vi "DataTranslation_server.vi"(0 "Board type":T1=enum."DT LV-link", 1 "interval scanning":bool, 2 "Client Time":dbl=3399992102.447224, 5 "No of samples+extra":i32=200 min=0 step=1, 7 "Trigger mode":T2, 9 "output polarity":u16(ring)=1 items=["do not change", "positive", "negative"], 11 "Ch & spans":T3[](array[typedef])=[{"high limit (10V)"=10.0, "low limit (-10V)"=-10.0, "Ch No"=0, "Var name"="RV (Vin)", "Use Latest Calib"=FALSE}] {"low limit (-10V)" format="%.3f"; "high limit (10V)" format="%.3f"}, 12 "Actual Sampling rate (Hz)":dbl=10000.0 format="%.2f", 13 "Local Client?":bool=TRUE, 14 "Current Block No":i32) -> (4 "I16 data":i16[][](array[numeric]), 6 "Block Timings":T4={"Started"=3399991568.753699, "Ended"=3399991587.0837474, "Analogue Frequency Hz"=50000.0} {"Analogue Frequency Hz" format="%.2f"}, 10 "group channel settings":T5(array[cluster])=[{"channel"="", "upper input limits"=0.0, "lower input limits"=0.0, "range"=0.0, "polarity"=0, "gain"=0.0, "coupling"=0, "input mode"=0, "scale multiplier"=1.6666666666666668e-07, "scale offset"=0.0}] {"scale offset" format="%#_16f"; "scale multiplier" format="%#_16f"; "input mode" format="%#_16f"; "coupling" format="%#_16f"; "gain" format="%#_16f"; "polarity" format="%#_16f"; "range" format="%#_16f"; "lower input limits" format="%#_16f"; "upper input limits" format="%#_16f"}, 15 "error out":errorcluster={"status"=TRUE, "code"=1172, "source"="Error calling method LvLink2.LvTask.ReadDblData2DAs1D, (System.Reflection.TargetInvocationException: Exception has been thrown by the target of an invocation.\n\tInner Exception: LvLink2.LvException: Timeout) <append><b>LvLink2.LvException</b> in OLReadMultiple2D.vi->DataTranslation_server.vi->Acquire_Data.vi->Get_data.vi->Measurement.vi"})   [LabVIEW 2011]
uses:
  Controls/Block_start_and_end.ctl
  Controls/Ch_and_Spans.ctl
  Controls/Trigger_Mode.ctl
  Controls/Board_Types.ctl
  Data_Translation/DataTranslation_global.vi
  PWA/PWAtasksGLOBAL.vi
  <userlib>/LV-Link3/PolySubVIs/DtCreateAinChan.vi
  <userlib>/LV-Link3/PolySubVIs/DtOLTimingSetInput.vi
  Globals/Meas_global.vi
  <userlib>/LV-Link3/PolySubVIs/DtOLReadMultiple2D.vi
  <userlib>/LV-Link3/PolySubVIs/DtOLTriggerDigital.vi
panel:
  in  "error in":errorcluster
  out "AFG error out":errorcluster
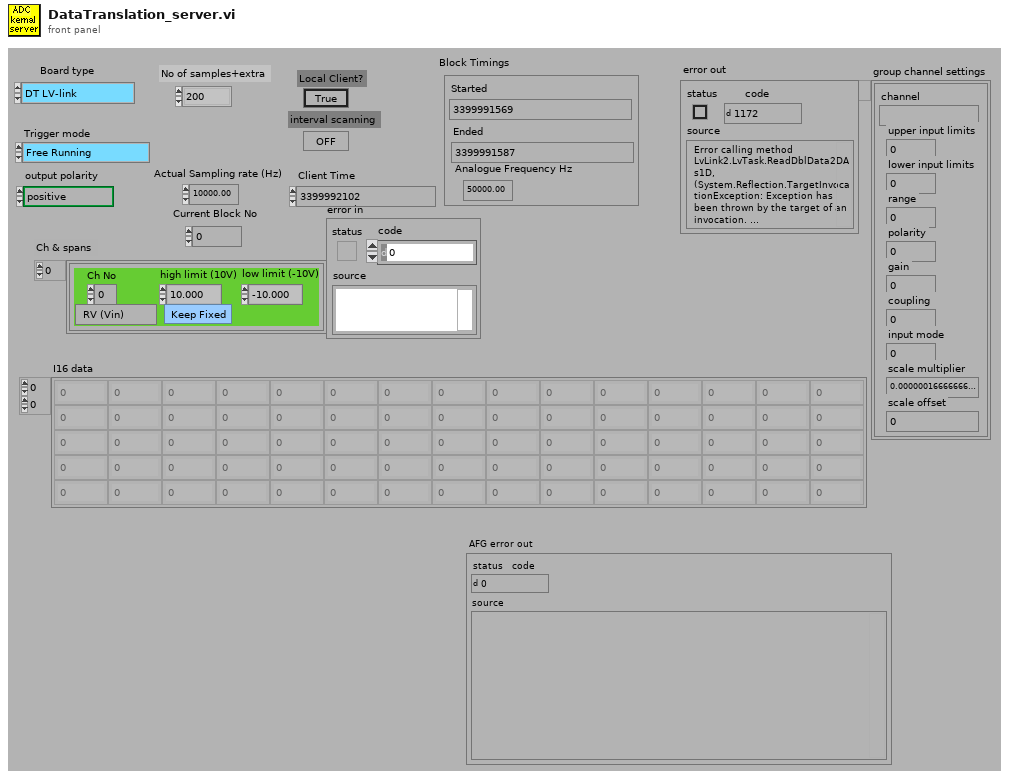
[diagram p1: front panel]
types:
  T1 = typedef "Board_Types.ctl" = enum16{"Simulate", "Local ADAM", "Server ADAM", "NI-DAQmx", "NI-DAQmxBase", "ADC488", "DT LV-link"}
  T2 = typedef "Trigger_Mode.ctl" = enum16{"Free Running", "Start on Trigger", "Trigger Every Block", "Trigger Every Sample"}
  T3 = typedef "Ch_and_Spans.ctl" = cluster{"high limit (10V)":sgl, "low limit (-10V)":sgl, "Ch No":i16, "Var name":string, "Use Latest Calib":bool}
  T4 = typedef "Block_start_and_end.ctl" = cluster{"Started":dbl, "Ended":dbl, "Analogue Frequency Hz":dbl}
  T5 = cluster{"channel":string, "upper input limits":sgl, "lower input limits":sgl, "range":sgl, "polarity":u16, "gain":sgl, "coupling":u16, "input mode":u16, "scale multiplier":dbl, "scale offset":dbl}[]
  T6 = cluster{"channel":string, "upper input limits":sgl, "lower input limits":sgl, "range":sgl, "polarity":u16, "gain":sgl, "coupling":u16, "input mode":u16, "scale multiplier":dbl, "scale offset":dbl}
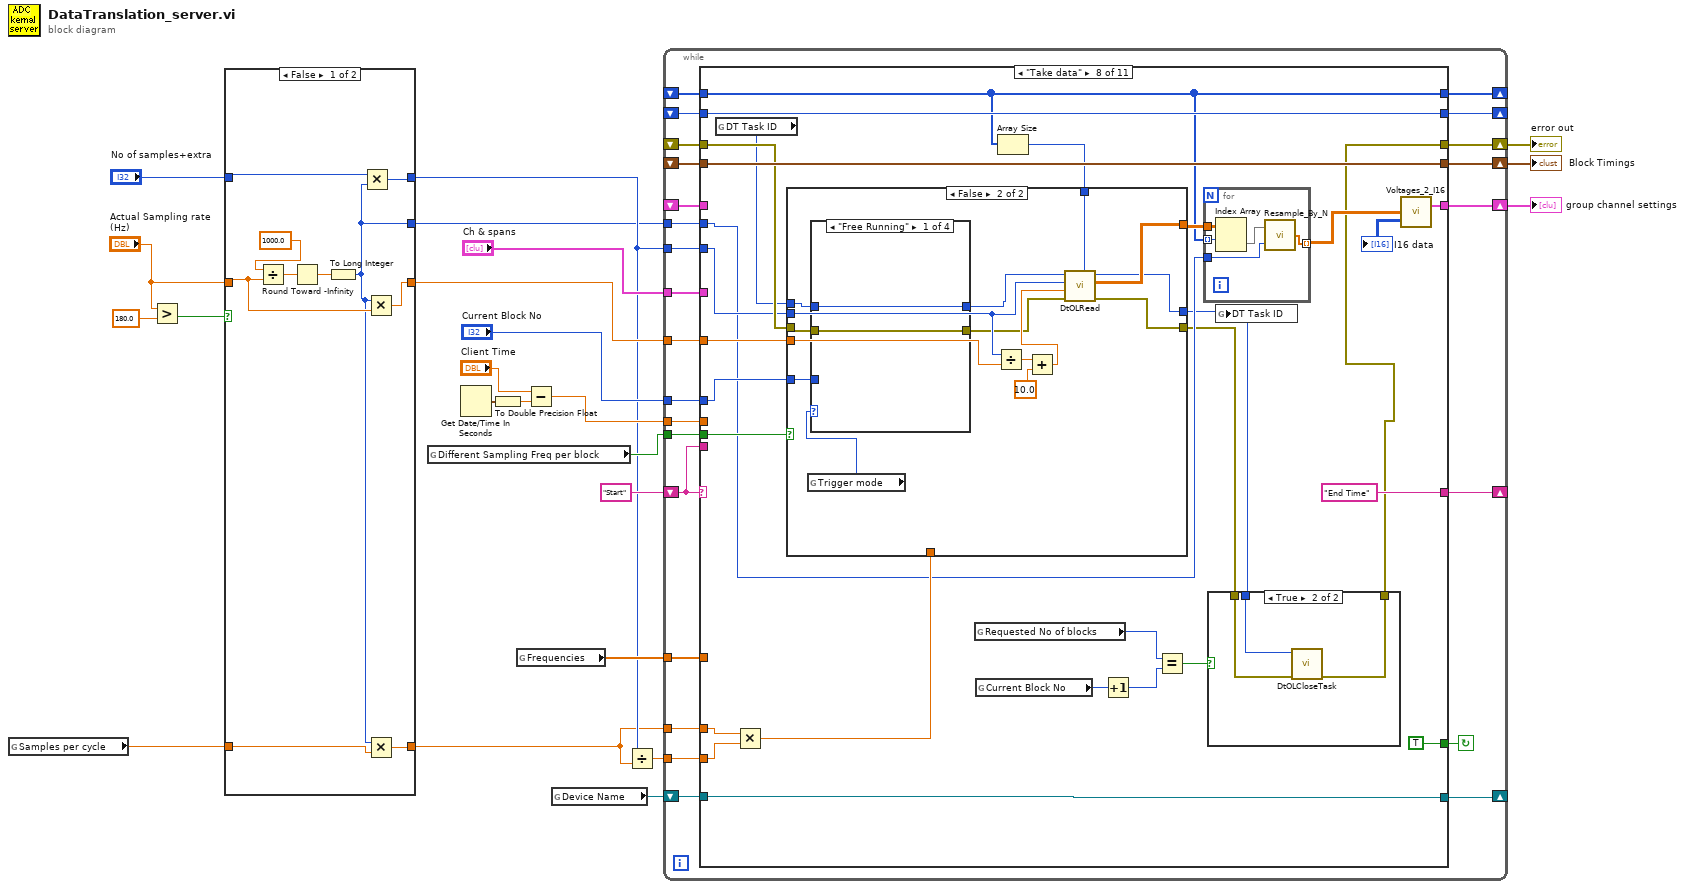
[diagram p0: block diagram]
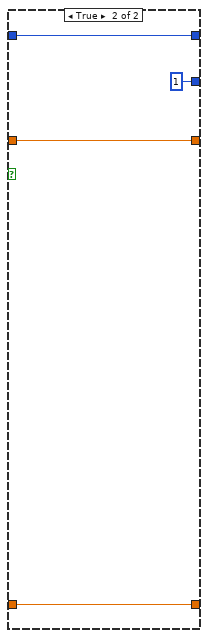
[diagram p2: hidden frame]
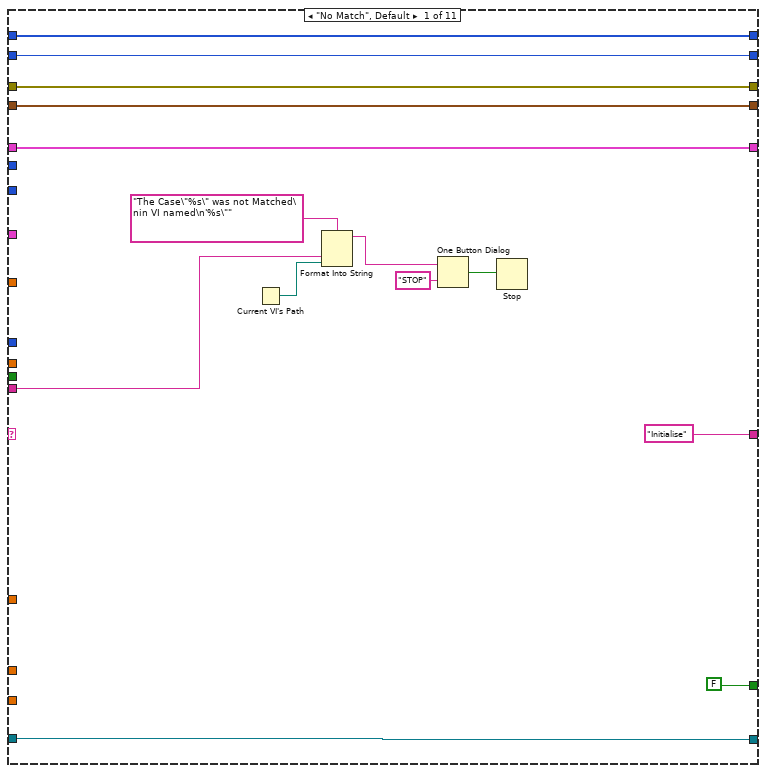
[diagram p3: hidden frame]
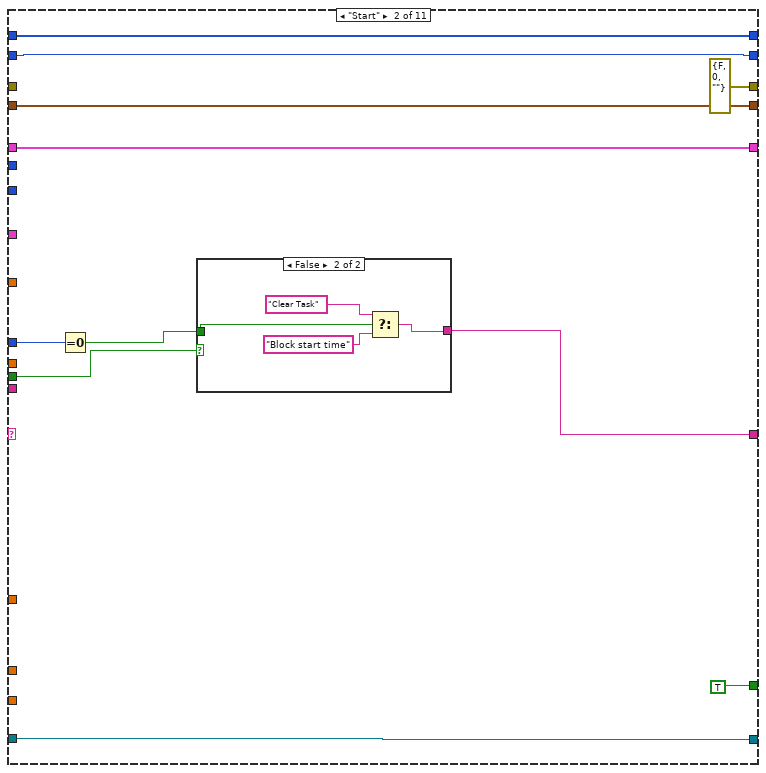
[diagram p4: hidden frame]
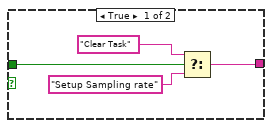
[diagram p5: hidden frame]
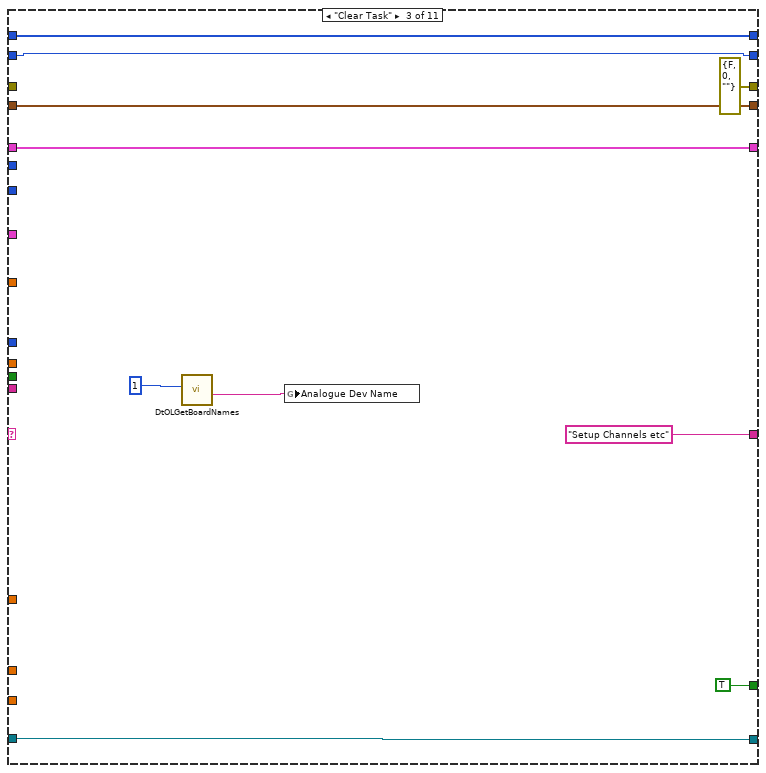
[diagram p6: hidden frame]
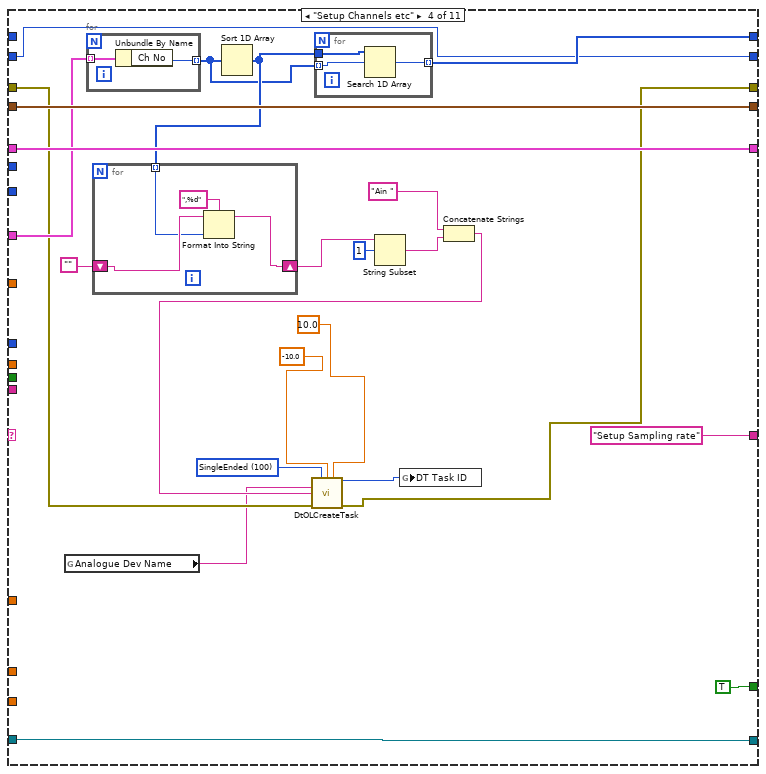
[diagram p7: hidden frame]
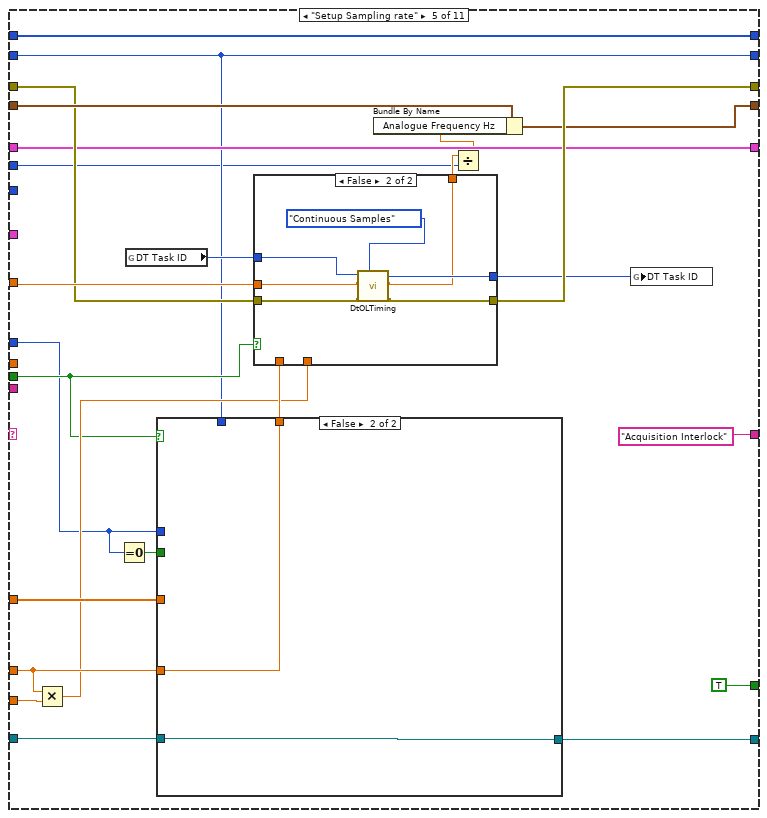
[diagram p8: hidden frame]
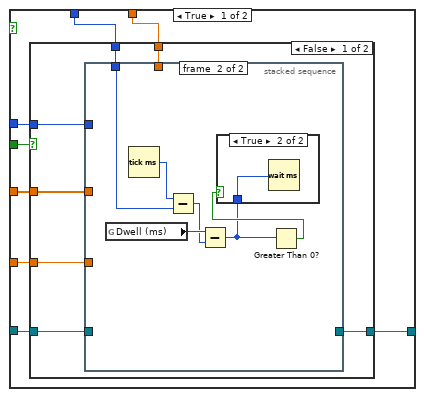
[diagram p9: hidden frame]
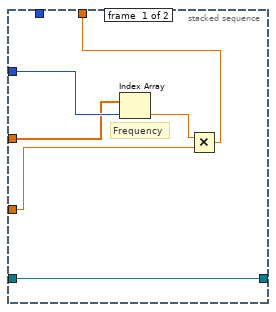
[diagram p10: hidden frame]
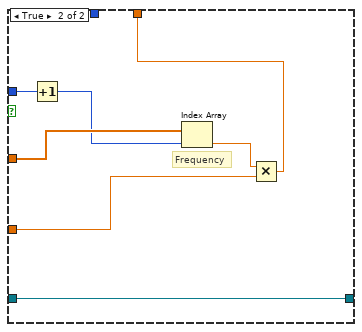
[diagram p12: hidden frame]
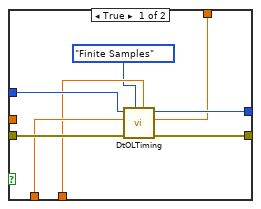
[diagram p13: hidden frame]
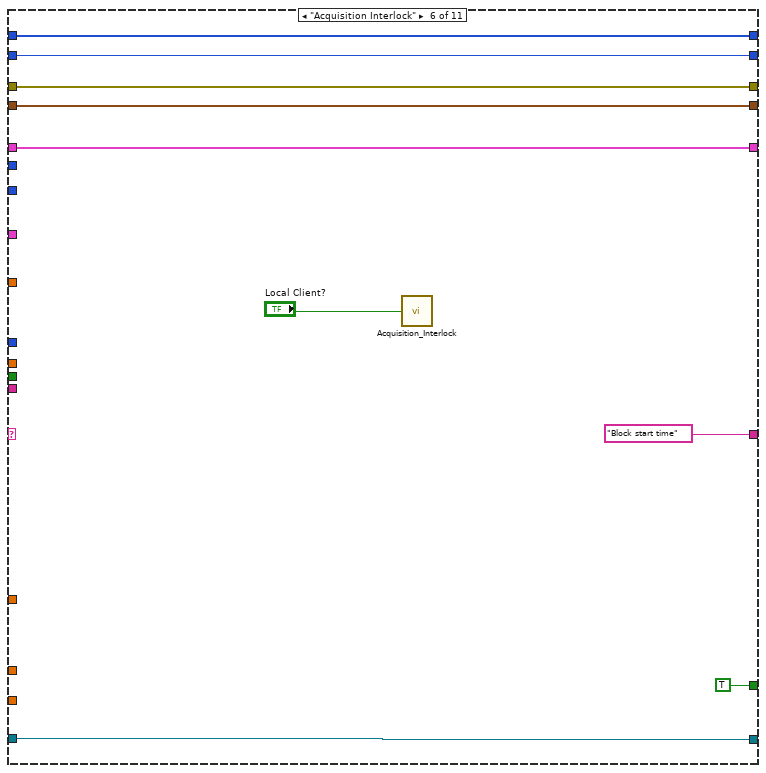
[diagram p14: hidden frame]
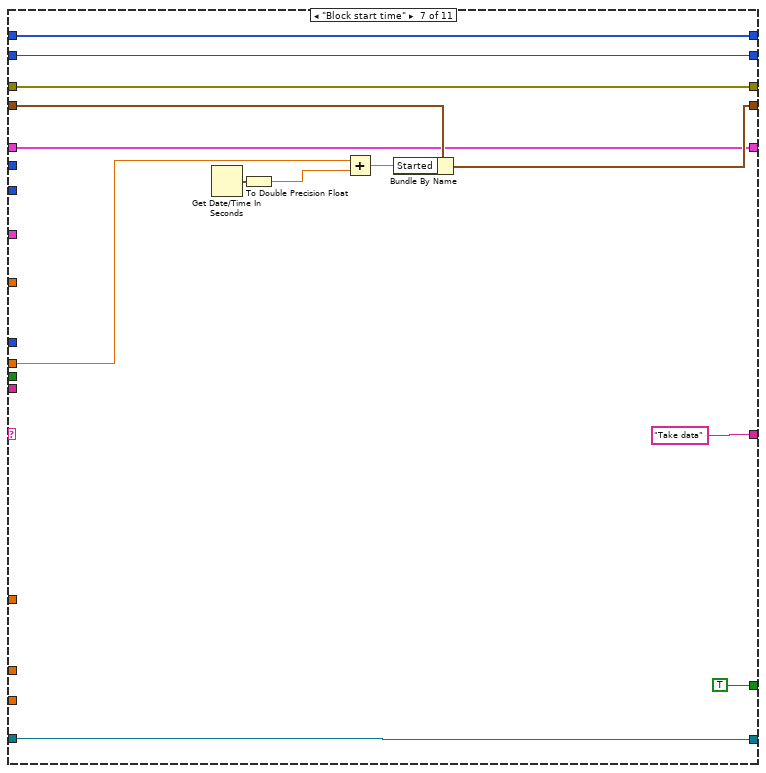
[diagram p15: hidden frame]
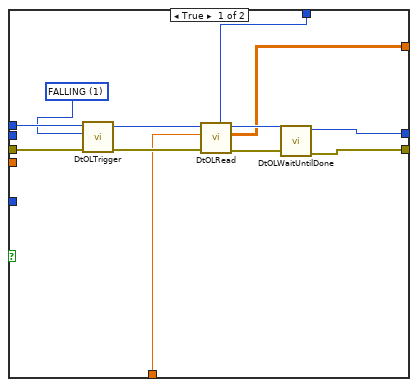
[diagram p17: hidden frame]
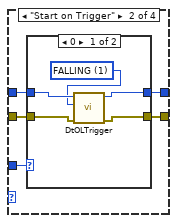
[diagram p18: hidden frame]
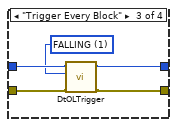
[diagram p20: hidden frame]
diagram:
  n1 = global read "DataTranslation_global.vi" "Samples per cycle"() -> (w2:dbl)
  n2 = Greater?(x="Actual Sampling rate (Hz)", y=180.0) -> (0:w8:bool)
  n3 = case shown="False" w8 {
    tunnel: "Actual Sampling rate (Hz)" -> [w27 w37]
    tunnel: [w28 w37] -> w6
    tunnel: [w30 w36] -> w5
    tunnel: "No of samples+extra" -> [w29 w36]
    tunnel: [w26 w35] -> w3
    tunnel: w2 -> [w25 w35]
    tunnel: [w24 1] -> w1
    frame False {
      n4 = Divide(x=1000.0, y=w27) -> (x/y=w32:dbl)
      n5 = Round Toward -Infinity(1:w32) -> (0:w31:dbl)
      n6 = To Long Integer(number=w31) -> (32bit integer=w24:i32)
      n7 = Multiply(x=w29, y=w24) -> (x*y=w30:i32)
      n8 = Multiply(x=w24, y=w27) -> (x*y=w28:dbl)
      n9 = Multiply(x=w24, y=w25) -> (x*y=w26:dbl)
    }
    frame True {
    }
  }
  n10 = global read "DataTranslation_global.vi" "Different Sampling Freq per block"() -> (w10:bool)
  n11 = Get Date/Time In Seconds() -> (seconds since 1Jan1904=w22:timestamp)
  n12 = To Double Precision Float(number=w22) -> (double precision float=w21:dbl)
  n13 = global read "DataTranslation_global.vi" "Frequencies"() -> (w11:dbl[])
  n14 = Subtract(x="Client Time", y=w21) -> (x-y=w19:dbl)
  n15 = global read "DataTranslation_global.vi" "Device Name"() -> (w12:refnum<visa-resource-name>)
  n16 = Divide(x=w5, y=w3) -> (x/y=w14:dbl)
  n17 = while {
    shift-left: "Start" -> [w60]
    shift-right: [w61] -> _
    shift-right: [w51] -> w16
    shift-left: _ -> [w59]
    shift-right: [w50] -> w17
    shift-left: _ -> [w58]
    tunnel: w19 -> [w57]
    tunnel: w6 -> [w56]
    tunnel: w5 -> [w55]
    tunnel: "Current Block No" -> [w54]
    tunnel: "Ch & spans" -> [w53]
    shift-right: [w49] -> w15
    shift-left: _ -> [w52]
    shift-right: [w48] -> _
    shift-left: _ -> [w47]
    tunnel: w3 -> [w45]
    shift-right: [w44] -> _
    shift-left: w12 -> [w46]
    tunnel: w14 -> [w43]
    tunnel: w10 -> [w42]
    tunnel: w11 -> [w41]
    shift-right: [w40] -> _
    shift-left: _ -> [w39]
    tunnel: w1 -> [w38]
    stop <- w62 continue-if-true
    n18 = case shown="\"Take data\"" w60 {
      tunnel: [FALSE TRUE TRUE TRUE TRUE TRUE TRUE TRUE w325 FALSE FALSE] -> w62
      tunnel: ["Initialise" w83 "Setup Channels etc" "Setup Sampling rate" "Acquisition Interlock" "Block start time" "Take data" "End Time" "Add info to block header" ("f") "End" ("f") "End" ("f")] -> w61
      tunnel: w60 -> [w71 _ _ _ _ _ _ _ _ _ _]
      tunnel: [w68 errorcluster {"status"=FALSE, "code"=0, "source"=""} ("error out") errorcluster {"status"=FALSE, "code"=0, "source"=""} ("error out") w108 w161 w221 w230 w237 w327 w352 w401] -> w51
      tunnel: w59 -> [w68 _ _ w109 w157 w221 w230 w259 w327 w352 w401]
      tunnel: [w66 w86 w104 w120 w158 w219 w234 w260 w332 w350 T4 {"Started"=0.0, "Ended"=0.0, "Analogue Frequency Hz"=1000.0} ("Block Timings")] -> w50
      tunnel: w58 -> [w66 w86 w104 w120 w159 w219 w235 w260 w333 w350 _]
      tunnel: w57 -> [_ _ _ _ _ _ w232 _ w324 _ _]
      tunnel: w56 -> [_ _ _ _ w160 _ _ w254 _ _ _]
      tunnel: w55 -> [_ _ _ _ _ _ _ w255 _ _ _]
      tunnel: w54 -> [_ w85 _ _ w142 _ _ w247 _ w338 _]
      tunnel: w53 -> [_ _ _ w119 _ _ _ _ _ _ _]
      tunnel: [w67 w82 w102 w126 w145 w218 w228 w261 w328 w348 w400] -> w49
      tunnel: w52 -> [w67 w82 w102 w126 w145 w218 w228 _ w328 w349 w400]
      tunnel: [w65 w80 w101 w116 w154 w217 w226 w246 w326 w351 w398] -> w48
      tunnel: w47 -> [w65 w80 w101 _ w154 w217 w226 w246 w326 w351 w398]
      tunnel: w46 -> [w64 w79 w100 w115 w151 w216 w225 w253 w323 w347 w397]
      tunnel: w41 -> [_ _ _ _ w153 _ _ _ _ w343 _]
      tunnel: w45 -> [_ _ _ _ w147 _ _ w251 _ _ _]
      tunnel: [w64 w79 w100 w115 w150 w216 w225 w253 w323 w346 w397] -> w44
      tunnel: w43 -> [_ _ _ _ w148 _ _ w252 _ _ _]
      tunnel: w42 -> [_ w78 _ _ w144 _ _ w249 w325 _ _]
      tunnel: [w63 w77 w99 w114 w143 w215 w224 w248 w322 w340 w396] -> w40
      tunnel: w39 -> [w63 w77 w99 w114 w143 w215 w224 w248 w322 _ w396]
      tunnel: w38 -> [_ _ _ _ w139 _ _ w244 _ _ _]
      frame "No Match", Default {
        n19 = Current VI's Path() -> (path=w70:path)
        n20 = Format Into String(format string="The Case\"%s\" was not Matched\nin VI named\n'%s\"" ("Format String"), w71, w70) -> (resulting string=w74:string)  [unwired: 2 in, 1 out]
        n21 = One Button Dialog(message=w74, button name ("OK")="STOP") -> (true=w72:bool)
        n22 = Stop(stop? (T)=w72) -> ()
      }
      frame "Start" {
        n23 = Equal To 0?(x=w85) -> (x = 0?=w84:bool)
        n24 = case shown="False" w78 {
          tunnel: w84 -> [w89 w93]
          tunnel: [w88 w92] -> w83
          frame True {
            n25 = Select(t="Clear Task", s=w89, f="Setup Sampling rate") -> (s? t:f=w88:string)
          }
          frame False {
            n26 = Select(t="Clear Task", s=w93, f="Block start time") -> (s? t:f=w92:string)
          }
        }
      }
      frame "Clear Task" {
        n27 = call <userlib>:"DtOLGetBoardNames.vi"("Select Board"=u32 1) -> ("Board Name"=w97:string)  [unwired: 8 in, 2 out]
        n28 = global write "PWAtasksGLOBAL.vi" "Analogue Dev Name"(w97) -> ()
      }
      frame "Setup Channels etc" {
        w110 = 100 items=["SingleEnded"=100, "Differential"=101] ("Channel Type")
        n29 = global read "PWAtasksGLOBAL.vi" "Analogue Dev Name"() -> (w106:string)
        n30 = for {
          tunnel: w119 -> [w133] mode=indexing
          tunnel: [w132] -> w117 mode=indexing
          n31 = Unbundle By Name(w133) -> ("Ch No"=w132:i16)
        }
        n32 = Sort 1D Array(array=w117) -> (sorted array=w118:i16[])
        n33 = for {
          shift-right: [w135] -> w125
          shift-left: "" -> [w136]
          tunnel: w118 -> [w134] mode=indexing
          n34 = Format Into String(format string=",%d", initial string=w136, w134) -> (resulting string=w135:string)  [unwired: 1 in, 1 out]
        }
        n35 = for {
          tunnel: w118 -> [w131]
          tunnel: w117 -> [w130] mode=indexing
          tunnel: [w129] -> w116 mode=indexing
          n36 = Search 1D Array(1D array=w131, element=w130) -> (index of element=w129:i32)  [unwired: 1 in]
        }
        n37 = String Subset(string=w125, offset (0)=1) -> (substring=w122:string)  [unwired: 1 in]
        n38 = Concatenate Strings("Ain ", w122) -> (w113:string)
        n39 = call-poly <userlib>:"DtOLCreateTask.vi"("Channel Type"=w110, "Range Min"=-10.0, "Range Max"=10.0, "Board Name"=w106, "Channel"=w113, "error in (no error)"=w109) -> ("Task out"=w107:i32, "error out"=w108:errorcluster)  [unwired: 7 in, 1 out]
        n40 = global write "DataTranslation_global.vi" "DT Task ID"(w107) -> ()
      }
      frame "Setup Sampling rate" {
        n41 = Multiply(x=w147, y=w148) -> (x*y=w146:dbl)
        n42 = Equal To 0?(x=w142) -> (x = 0?=w141:bool)
        n43 = global read "DataTranslation_global.vi" "DT Task ID"() -> (w155:i32)
        n44 = case shown="False" w144 {
          tunnel: w153 -> [w166 _]
          tunnel: [w170 w198] -> w152
          tunnel: w147 -> [w169 w198]
          tunnel: w142 -> [w168 _]
          tunnel: w151 -> [w167 w199]
          tunnel: [w165 w199] -> w150
          tunnel: w143 -> [w164 _]
          tunnel: w141 -> [w163 _]
          frame True {
            n45 = case shown="False" w163 {
              tunnel: [w177 w194] -> w170
              tunnel: w169 -> [w176 w193]
              tunnel: w168 -> [w171 w195]
              tunnel: w167 -> [w175 w192]
              tunnel: w166 -> [w174 w196]
              tunnel: [w173 w192] -> w165
              tunnel: w164 -> [w172 _]
              frame False {
                n46 = stacked-sequence {
                  tunnel: [w183 _] -> w177
                  tunnel: w176 -> [w182 _]
                  tunnel: w171 -> [w181 _]
                  tunnel: w175 -> [w178 _]
                  tunnel: w174 -> [w180 _]
                  tunnel: [w178 _] -> w173
                  tunnel: w172 -> [_ w188]
                  frame #0 {
                    # "Frequency"
                    n47 = Index Array(array=w180, index=w181) -> (element=w179:dbl)
                    n48 = Multiply(x=w179, y=w182) -> (x*y=w183:dbl)
                  }
                  frame #1 {
                    n49 = global read "DataTranslation_global.vi" "Dwell (ms)"() -> (w187:u32)
                    n50 = Tick Count (ms)() -> (millisecond timer value=w189:u32)
                    n51 = Subtract(x=w189, y=w188) -> (x-y=w186:u32)
                    n52 = Subtract(x=w187, y=w186) -> (x-y=w184:u32)
                    n53 = Greater Than 0?(x=w184) -> (x > 0?=w185:bool)
                    n54 = case shown="True" w185 {
                      tunnel: w184 -> [_ w190]
                      frame False {
                      }
                      frame True {
                        n55 = Wait (ms)(milliseconds to wait=w190) -> ()  [unwired: 1 out]
                      }
                    }
                  }
                }
              }
              frame True {
                # "Frequency"
                n56 = Increment(x=w195) -> (x+1=w191:i32)
                n57 = Index Array(array=w196, index=w191) -> (element=w197:dbl)
                n58 = Multiply(x=w197, y=w193) -> (x*y=w194:dbl)
              }
            }
          }
          frame False {
          }
        }
        n59 = case shown="False" w144 {
          tunnel: [w204 w209] -> w161
          tunnel: w160 -> [_ w212]
          tunnel: [w203 w211] -> w140
          tunnel: w157 -> [w205 w210]
          tunnel: [w206 w214] -> w156
          tunnel: w155 -> [w207 w213]
          tunnel: w152 -> [w202 _]
          tunnel: w146 -> [w201 _]
          frame True {
            n60 = call-poly <userlib>:"DtOLTiming.vi"("Samples Per Channel"=w201, "Sample Mode"=enum16{"Finite Samples", "Continuous Samples"}."Finite Samples", "error in (no error)"=w205, "Sample Freq (Hz)"=w202, "Task in"=w207) -> ("error out"=w204:errorcluster, "Actual Sample Freq"=w203:dbl, "Task out"=w206:i32)  [unwired: 3 in, 1 out]
          }
          frame False {
            n61 = call-poly <userlib>:"DtOLTiming.vi"("Sample Mode"=enum16{"Finite Samples", "Continuous Samples"}."Continuous Samples", "error in (no error)"=w210, "Sample Freq (Hz)"=w212, "Task in"=w213) -> ("error out"=w209:errorcluster, "Actual Sample Freq"=w211:dbl, "Task out"=w214:i32)  [unwired: 4 in, 1 out]
          }
        }
        n62 = Divide(x=w140, y=w139) -> (x/y=w138:dbl)
        n63 = Bundle By Name(cluster=w159, "Analogue Frequency Hz"=w138) -> (w158:T4)
        n64 = global write "DataTranslation_global.vi" "DT Task ID"(w156) -> ()
      }
      frame "Acquisition Interlock" {
        n65 = call "Acquisition_Interlock.vi"("Local Control"="Local Client?") -> ()
      }
      frame "Block start time" {
        n66 = Get Date/Time In Seconds() -> (seconds since 1Jan1904=w236:timestamp)
        n67 = To Double Precision Float(number=w236) -> (double precision float=w233:dbl)
        n68 = Add(x=w232, y=w233) -> (x+y=w231:dbl)
        n69 = Bundle By Name(cluster=w235, "Started"=w231) -> (w234:T4)
      }
      frame "Take data" {
        n70 = global read "DataTranslation_global.vi" "DT Task ID"() -> (w258:i32)
        n71 = Multiply(x=w251, y=w252) -> (x*y=w250:dbl)
        n72 = global read "Meas_global.vi" "Requested No of blocks"() -> (w241:i32)
        n73 = global read "Meas_global.vi" "Current Block No"() -> (w243:i32)
        n74 = Array Size(array=w246) -> (size(s)=w245:i32)
        n75 = case shown="False" w249 {
          tunnel: w259 -> [w280 w290]
          tunnel: [w277 w284] -> w238
          tunnel: [w274 w282] -> w240
          tunnel: w258 -> [w273 w291]
          tunnel: [w271 w283] -> w257
          tunnel: w255 -> [_ w287]
          tunnel: w254 -> [_ w295]
          tunnel: w250 -> [w270 _]
          tunnel: w247 -> [_ w289]
          tunnel: w245 -> [w269 w281]
          frame True {
            w272 = 1 items=["RISING", "FALLING"] ("External Trigger Polarity")
            n76 = call-poly <userlib>:"DtOLTrigger.vi"("error in (no error)"=w280, "External Trigger Polarity"=w272, "Task in"=w273) -> ("error out"=w279:errorcluster, "Task out"=w276:i32)  [unwired: 7 in]
            n77 = call-poly <userlib>:"DtOLRead.vi"("Number Chan to Read"=w269, "error in (no error)"=w279, "Samples Per Channel"=w270, "Task in"=w276) -> ("error out"=w278:errorcluster, "2D Data out"=w271:dbl[][], "Task out"=w275:i32)  [unwired: 3 in, 2 out]
            n78 = call <userlib>:"DtOLWaitUntilDone.vi"("error in"=w278, "Task in"=w275) -> ("error out"=w277:errorcluster, "Task out"=w274:i32)  [unwired: 8 in]
          }
          frame False {
            n79 = global read "Meas_global.vi" "Trigger mode"() -> (w292:T2)
            n80 = case shown="\"Free Running\"" w292 {
              tunnel: [w297 w299 w313 w316] -> w288
              tunnel: w291 -> [w297 w301 w314 w316]
              tunnel: [w296 w298 w310 w315] -> w285
              tunnel: w290 -> [w296 w300 w311 w315]
              tunnel: w289 -> [_ w302 _ _]
              frame "Free Running" {
              }
              frame "Start on Trigger" {
                n81 = case shown="0" w302 {
                  tunnel: w301 -> [w307 w309]
                  tunnel: w300 -> [w305 w308]
                  tunnel: [w303 w309] -> w299
                  tunnel: [w304 w308] -> w298
                  frame 0 {
                    w306 = 1 items=["RISING", "FALLING"] ("External Trigger Polarity")
                    n82 = call-poly <userlib>:"DtOLTrigger.vi"("error in (no error)"=w305, "External Trigger Polarity"=w306, "Task in"=w307) -> ("error out"=w304:errorcluster, "Task out"=w303:i32)  [unwired: 7 in]
                  }
                  frame 1, Default {
                  }
                }
              }
              frame "Trigger Every Block" {
                w312 = 1 items=["RISING", "FALLING"] ("External Trigger Polarity")
                n83 = call-poly <userlib>:"DtOLTrigger.vi"("error in (no error)"=w311, "External Trigger Polarity"=w312, "Task in"=w314) -> ("error out"=w310:errorcluster, "Task out"=w313:i32)  [unwired: 7 in]
              }
              frame "Trigger Every Sample" {
              }
            }
            n84 = Divide(x=w287, y=w295) -> (x/y=w293:dbl)
            n85 = Add(x=w293, y=10.0) -> (x+y=w286:dbl)
            n86 = call-poly <userlib>:"DtOLRead.vi"("Number Chan to Read"=w281, "error in (no error)"=w285, "Timeout"=w286, "Samples Per Channel"=w287, "Task in"=w288) -> ("error out"=w284:errorcluster, "2D Data out"=w283:dbl[][], "Task out"=w282:i32)  [unwired: 2 in, 2 out]
          }
        }
        n87 = Increment(x=w243) -> (x+1=w242:i32)
        n88 = Equal?(x=w241, y=w242) -> (x = y?=w239:bool)
        n89 = for {
          tunnel: w246 -> [w321] mode=indexing
          tunnel: w257 -> [w320]
          tunnel: [w318] -> w256 mode=indexing
          tunnel: w244 -> [w317]
          n90 = Index Array(array=w320, index (row)=w321) -> (element=w319:dbl[])  [unwired: 1 in]
          n91 = call "Resample_By_N.vi"("Resample Factor"=w317, "Array In"=w319) -> ("Array Out"=w318:dbl[])
        }
        n92 = case shown="True" w239 {
          tunnel: w240 -> [_ w268]
          tunnel: w238 -> [w265 w267]
          tunnel: [w265 w266] -> w237
          frame False {
          }
          frame True {
            n93 = call <userlib>:"DtOLCloseTask.vi"("Error in"=w267, "Task in"=w268) -> ("Error Out"=w266:errorcluster)  [unwired: 9 in]
          }
        }
        n94 = global write "DataTranslation_global.vi" "DT Task ID"(w240) -> ()
        n95 = call "Voltages_2_I16.vi"("Voltages"=w256) -> ("Group Channel Settings"=w261:T5, "I16 data"=→"I16 data":i16[][])
      }
      frame "End Time" {
        # "Final transpose to get 2D data output correctly"
        n96 = Get Date/Time In Seconds() -> (seconds since 1Jan1904=w334:timestamp)
        n97 = To Double Precision Float(number=w334) -> (double precision float=w331:dbl)
        n98 = Add(x=w324, y=w331) -> (x+y=w330:dbl)
        n99 = Bundle By Name(cluster=w333, "Ended"=w330) -> (w332:T4)
      }
      frame "Add info to block header" {
        n100 = global read "Meas_global.vi" "Requested No of blocks"() -> (w341:i32)
        n101 = global read "DataTranslation_global.vi" "Amplitudes"() -> (w335:dbl[])
        n102 = Index Array(array=w335, index=w338) -> (element=w345:dbl)
        n103 = Index Array(array=w343, index=w338) -> (element=w344:dbl)
        n104 = Decrement(x=w341) -> (x-1=w339:i32)
        n105 = for {
          tunnel: w349 -> [w383] mode=indexing
          tunnel: [w382] -> w348 mode=indexing
          tunnel: w345 -> [w381]
          tunnel: w344 -> [w380]
          i -> [w384]
          n106 = case shown="0" w384 {
            tunnel: w383 -> [w394 w395]
            tunnel: [w388 w395] -> w382
            tunnel: w381 -> [w391 _]
            tunnel: w380 -> [w390 _]
            frame 0 {
              n107 = call "Value_to_string.vi"("Value"=w391, "Label for value"="Function_Generator_Amplitude") -> ("Output string"=w387:string)  [unwired: 1 in]
              n108 = call "Value_to_string.vi"("precision"="0", "Value"=w390, "Label for value"="Function_Generator_Frequency") -> ("Output string"=w386:string)
              n109 = Concatenate Strings(w387, w386) -> (w385:string)
              n110 = Bundle By Name(cluster=w394, "channel"=w385) -> (w388:T6)
            }
            frame 1, Default {
            }
          }
        }
        n111 = Equal?(x=w338, y=w339) -> (x = y?=w342:bool)
        n112 = case shown="False" w342 {
          tunnel: w347 -> [w367 w377]
          tunnel: [w358 w375] -> w346
          tunnel: [w360 w376] -> w336
          tunnel: w343 -> [w363 w378]
          tunnel: w335 -> [w364 w379]
          tunnel: w338 -> [w362 _]
          tunnel: [w364 w379] -> _
          tunnel: [w363 w378] -> _
          tunnel: "error in" -> [w355 w373]
          frame False {
            w368 = "SOUR1" ("input 1")
            w371 = ":%s:FREQ %.;%g;"  # Frequency Command
            w372 = ":%s:VOLT %.;%g;"  # Amplitude Command
            n113 = Increment(x=w362) -> (x+1=w361:i32)
            n114 = Index Array(array=w364, index=w361) -> (element=w366:dbl)
            n115 = Index Array(array=w363, index=w361) -> (element=w365:dbl)
            n116 = Format Into String(format string=w371, w368, w365) -> (resulting string=w369:string)  [unwired: 2 in, 1 out]
            n117 = Format Into String(format string=w372, initial string=w369, w368, w366) -> (resulting string=w370:string)  [unwired: 1 in, 1 out]
            n118 = VISA Write(VISA resource name=w367, write buffer=w370, error in (no error)=w355) -> (VISA resource name out=w359:refnum<visa-resource-name>, error out=w357:errorcluster)  [unwired: 1 out]
            n119 = VISA Write(VISA resource name=w359, write buffer="OUTP1:STAT ON", error in (no error)=w357) -> (VISA resource name out=w358:refnum<visa-resource-name>, error out=w360:errorcluster)  [unwired: 1 out]
          }
          frame True {
            n120 = VISA Write(VISA resource name=w377, write buffer="OUTP1:STAT OFF", error in (no error)=w373) -> (VISA resource name out=w375:refnum<visa-resource-name>, error out=w376:errorcluster)  [unwired: 1 out]
          }
        }
        "AFG error out" <- w336
        n121 = Tick Count (ms)() -> (millisecond timer value=w340:u32)
      }
      frame "Extra case" {
      }
    }
  }
  "Block Timings" <- w17
  "error out" <- w16
  "group channel settings" <- w15
